vi "Actor Core.vi"(8 "error in":errorcluster, 11 "MockModel in":refnum<class "TestModelFastPublish.lvclass">) -> (0 "error out":errorcluster, 3 "Actor out":refnum<class "Actor.lvclass">)   [LabVIEW 2015, in "TestModels.lvlib" / "TestModelFastPublish.lvclass"]
doc: "(<B>Filename</B>: Actor Framework.lvlib:Actor.lvclass:Actor Core.vi)\n\nReceives messages to the actor, reacts to them, and initiates any error handling that may shut the actor down.\n\nDescendant classes may override this VI to append parallel tasks for the actor to complete while it handles messages. Overrides use the Call Parent Method node."
uses:
  TestModelFastPublish.lvclass
  <vilib>/ActorFramework/Actor/Actor.lvclass
  <vilib>/Platform/TimedLoop/XDataNode/wakeup.ctl
  Framework/IModel/IModel/IModel.lvclass/IModel.ctl
  Framework/AbstractMessages/PreAddressedMsg/PreAddressedMsg.lvclass/PreAddressedMsg.ctl
  Framework/IMediator/IMediator Messages/Publish Msg/Publish Msg.lvclass/Publish Msg.ctl
  <vilib>/ActorFramework/Message Enqueuer/Message Enqueuer.lvclass/Message Enqueuer.ctl
  Framework/IMediator/IMediator Messages/Publish Msg/Send Pre-Addressed Publish.vi
  <vilib>/ActorFramework/Message Enqueuer/Enqueue.vi
  Framework/AbstractMessages/PreAddressedMsg/Read Return Address.vi
  <vilib>/ActorFramework/Message Priority Queue/Priority Enqueue.vi
  Framework/IModel/IModel/IModel.lvclass
  <vilib>/Platform/TimedLoop/XDataNode/XDNodeRunTimeDep.lvlib
panel:
  in  "Stop Publisher":bool
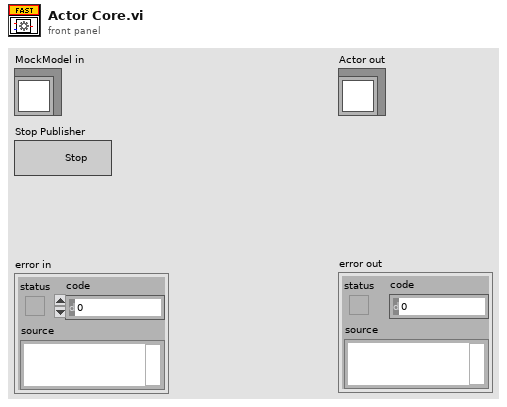
[diagram p1: front panel]
types:
  T1 = typedef "XDNodeRunTimeDep.lvlib/wakeup.ctl" = enum32{"Normal", "Aborted", "Asynchronous wakeup", "Timing source error", "Timed loop error", "Timeout"}
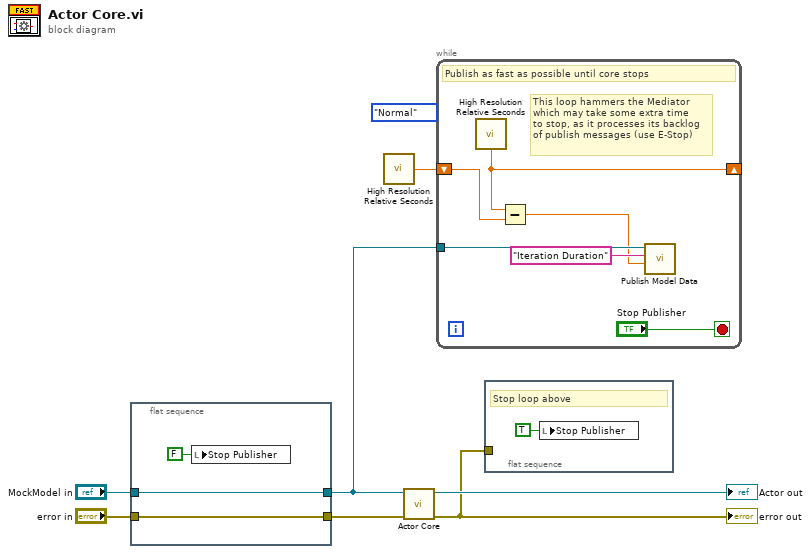
[diagram p0: block diagram]
diagram:
  n1 = flat-sequence {
    tunnel: "error in" -> [w10]
    tunnel: [w10] -> w4
    tunnel: "MockModel in" -> [w9]
    tunnel: [w9] -> w2
    frame #0 {
      n2 = local write "Stop Publisher"(FALSE ("Stop Publisher")) -> ()
    }
  }
  n3 = call <vilib>:"High Resolution Relative Seconds.vi"() -> ("relative seconds"=w1:dbl)
  n4 = call-parent "Actor Core.vi"("error in"=w4, "Actor in"=w2) -> ("error out"=w5:errorcluster, "Actor out"=→"Actor out":refnum<class "Actor.lvclass">)  [unwired: 8 in]
  "error out" <- w5
  n5 = while {
    tunnel: w2 -> [w15]
    shift-right: [w12] -> _
    shift-left: w1 -> [w13]
    stop <- "Stop Publisher" stop-if-true
    (unwired) wakeup."Normal" ("Wakeup Reason")
    (unwired) wakeup."Normal" ("Wakeup Reason")
    # "This loop hammers the Mediator\nwhich may take some extra time\nto stop, as it processes its backlog\nof publish messages (use E-Stop)"
    # "Publish as fast as possible until core stops"
    n6 = call <vilib>:"High Resolution Relative Seconds.vi"() -> ("relative seconds"=w12:dbl)
    n7 = Subtract(x=w12, y=w13) -> (x-y=w11:dbl)
    n8 = call "Publish Model Data.vi"("Data to Publish"=w11, "Datum Name"="Iteration Duration" ("Topic Name"), "IModel in"=w15) -> ()  [unwired: 7 in, 2 out]
  }
  n9 = flat-sequence {
    tunnel: w5 -> [_]
    frame #0 {
      # "Stop loop above"
      n10 = local write "Stop Publisher"(TRUE ("Stop Publisher")) -> ()
    }
  }
